vi "FTW-Messenger-Destroy.vi"(0 "Messenger":refnum<class "FTW-Messenger-Actor.lvclass">, 11 "error in":errorcluster) -> (15 "error out":errorcluster)   [LabVIEW 2014, in "FTW-Messenger-Actor.lvclass"]
uses:
  FTW-Messenger-Actor.lvclass
  Messenger/FTW-Messenger.lvclass
panel:
  # "Inputs"
  # "Outputs"
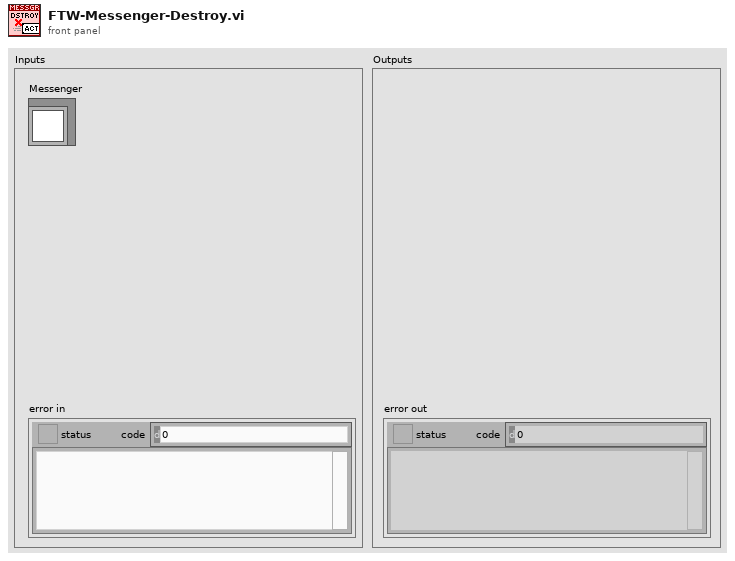
[diagram p1: front panel]
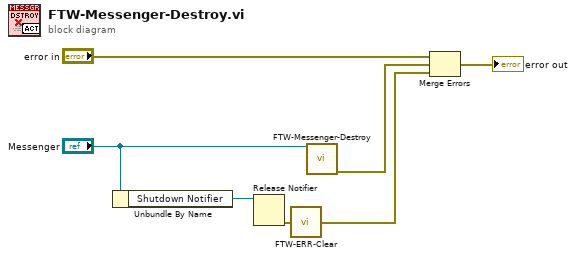
[diagram p0: block diagram]
diagram:
  n1 = Unbundle By Name("Messenger") -> ("Shutdown Notifier"=w6:refnum<notifier>)
  n2 = Release Notifier(notifier=w6) -> (error out=w2:errorcluster)  [unwired: 2 in, 2 out]
  n3 = call "FTW-ERR-Clear.vi"("error to snuff"=w2) -> ("no error"=w1:errorcluster)
  n4 = call-parent "FTW-Messenger-Destroy.vi"("Messenger"="Messenger") -> ("error out"=w3:errorcluster)  [unwired: 14 in]
  n5 = Merge Errors("error in", w3, w1) -> (→"error out":errorcluster)
